vi "PageEngine.vi"() -> ()   [LabVIEW 2016, in "PCM PanelSplit.lvclass"]
uses:
  PCM PanelSplit.lvclass
  <vilib>/Utility/error.llb/DialogType.ctl
  PanelSplitToolkit/QueueManager.llb/CreatQueue.vi
  PanelSplitToolkit/QueueManager.llb/Remove.vi
  PanelSplitToolkit/QueueManager.llb/Insert.vi
  PanelSplitToolkit/QueueManager.llb/Destroy.vi
  PanelSplitToolkit/PanelRootNode/PanelRootNode.lvclass
panel:
  in  "Parameters":T1
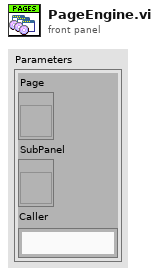
[diagram p1: front panel]
types:
  T1 = cluster{"Page":refnum<vi>, "SubPanel":refnum<vi>, "Caller":string}
  T2 = cluster{"error":errorcluster, "Event":string, "Data":variant, "Q_Local":string, "DyPageNames":string[], "DyPageVIRefs":refnum<vi>[], "PageTreeTags":string[], "CurrentPage":string, "PageVIPath":path, "PanelUIQName":string, "Send":cluster{"VI*ToSend":refnum<vi>, "EventToSend":string, "DataToSend":variant}, "PageCtr*":refnum<vi>, "SubPanel*":refnum<vi>, "Q_Caller":string, "FixedPages":cluster{"FixedPageNames":string[], "FixedPageVIRefs":refnum<vi>[]}}
  T3 = cluster{"Page":refnum<vi>, "SubPanel":refnum<vi>}
  T4 = typedef "DialogType.ctl" = u16
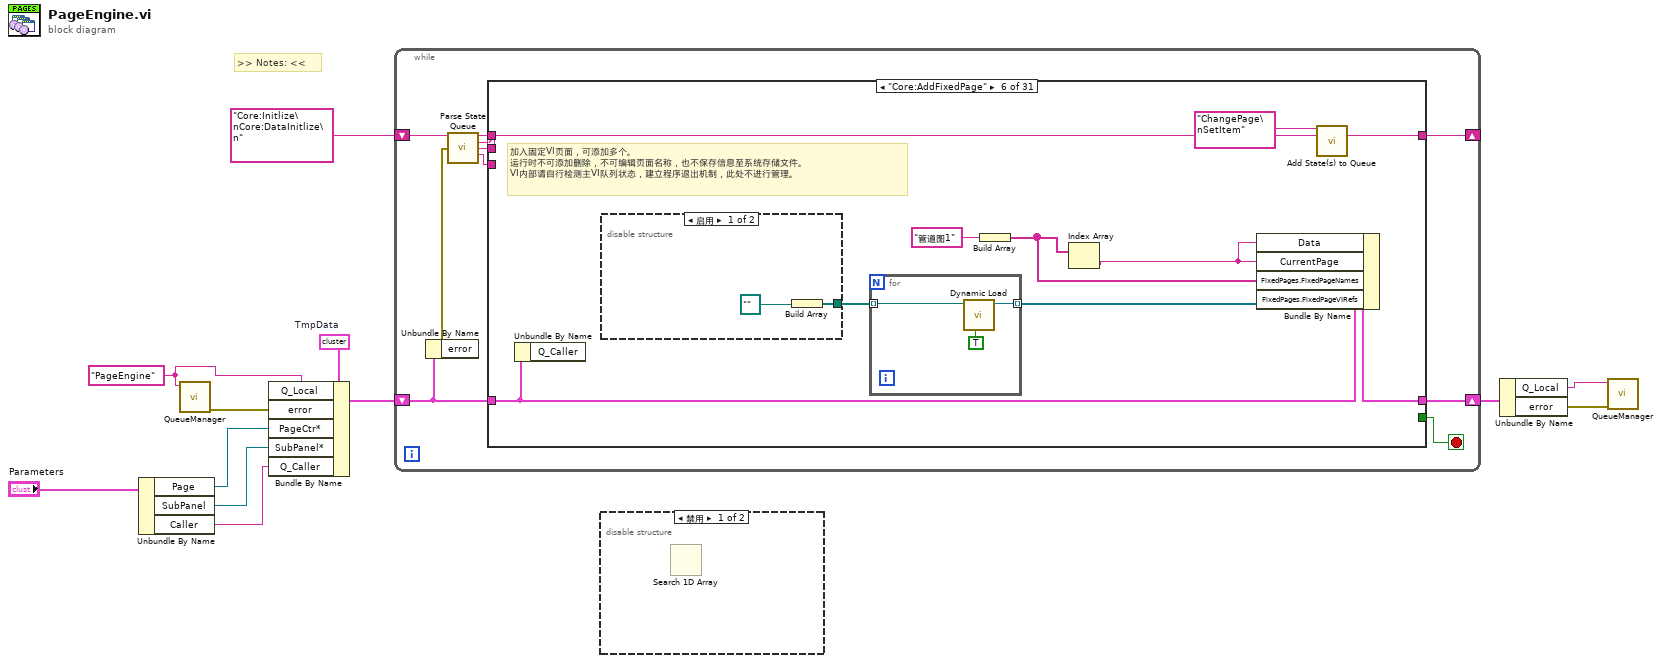
[diagram p0: block diagram]
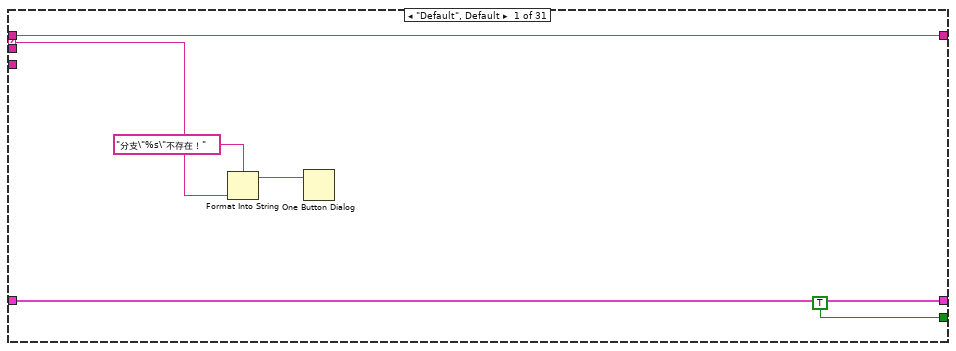
[diagram p3: hidden frame]
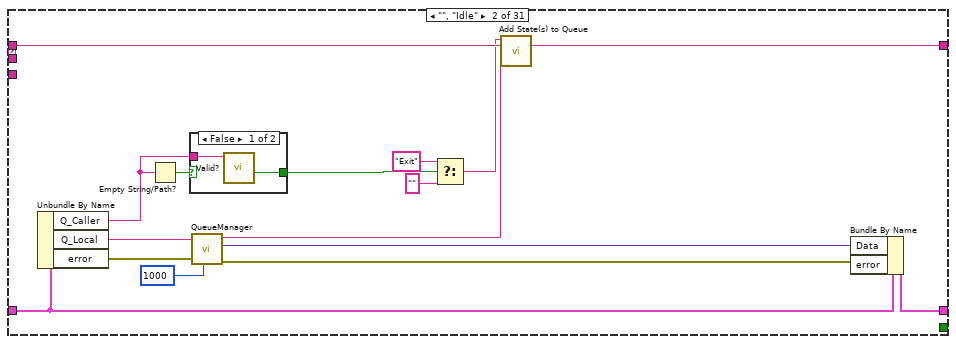
[diagram p4: hidden frame]
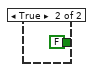
[diagram p5: hidden frame]
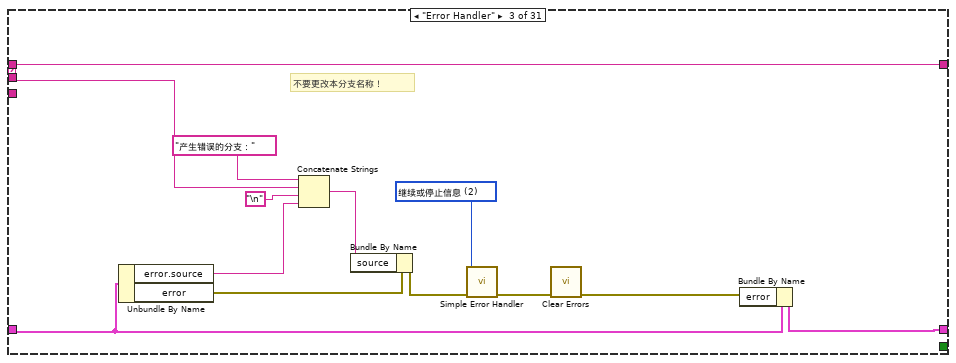
[diagram p6: hidden frame]
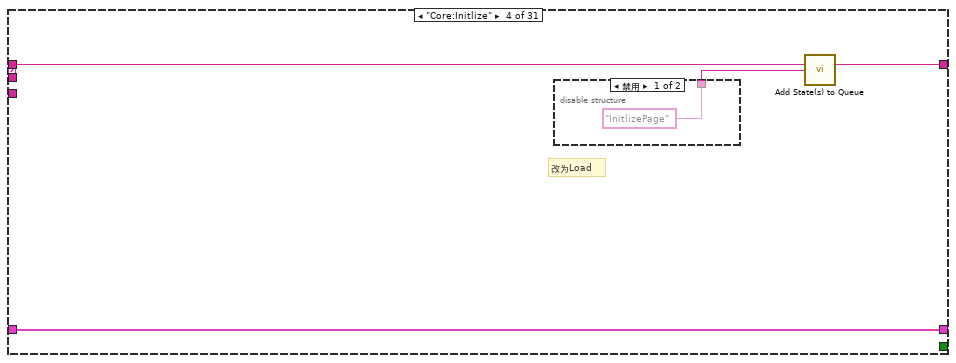
[diagram p7: hidden frame]
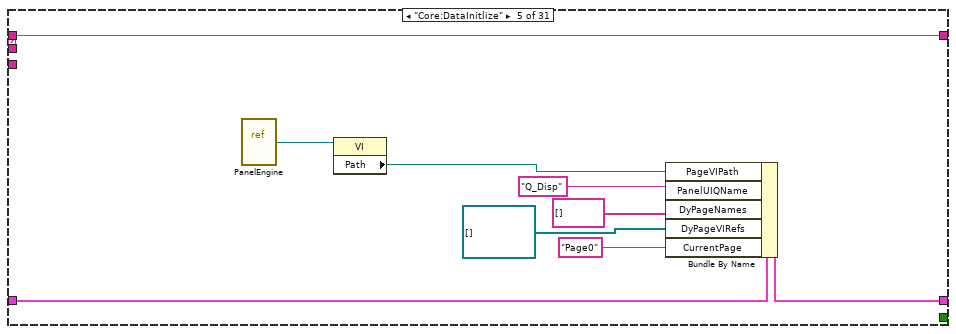
[diagram p9: hidden frame]
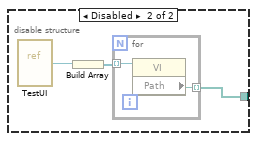
[diagram p10: hidden frame]
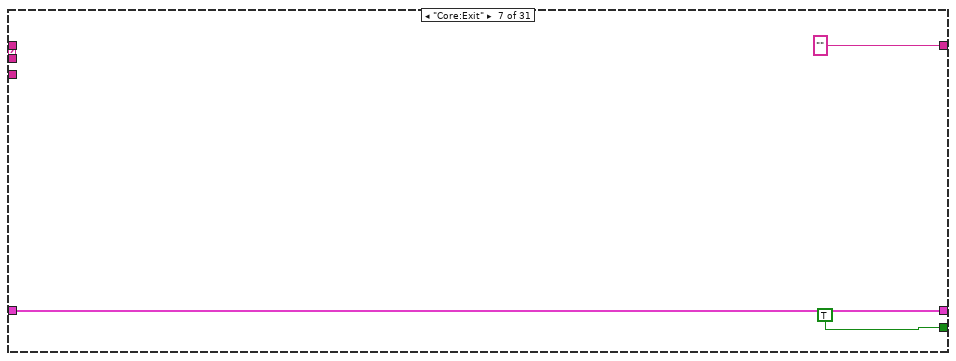
[diagram p11: hidden frame]
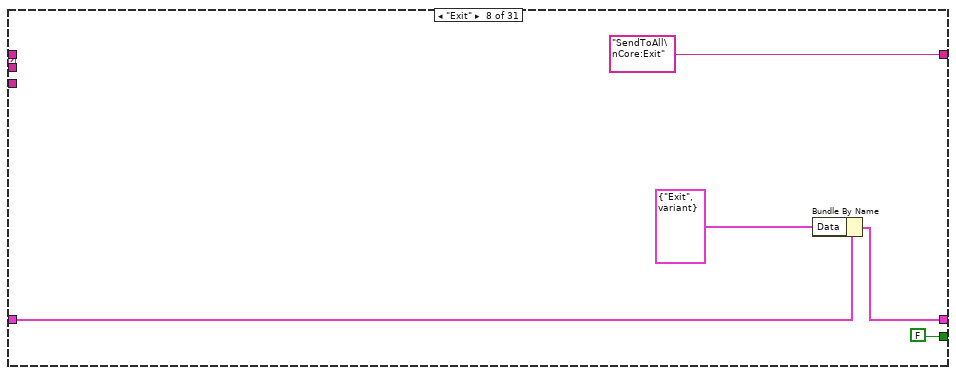
[diagram p12: hidden frame]
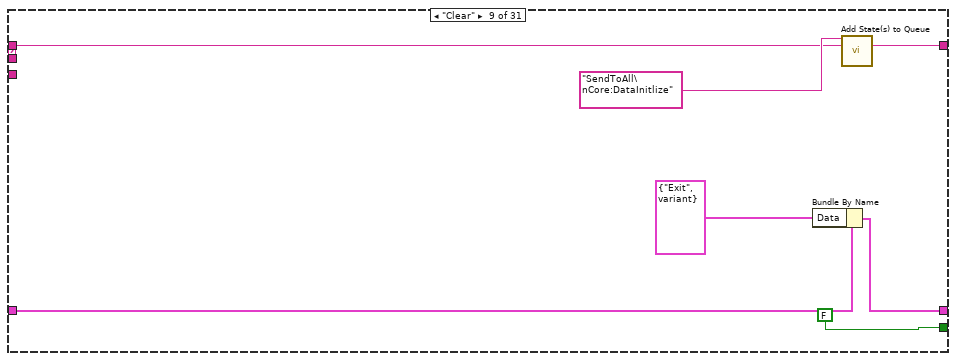
[diagram p13: hidden frame]
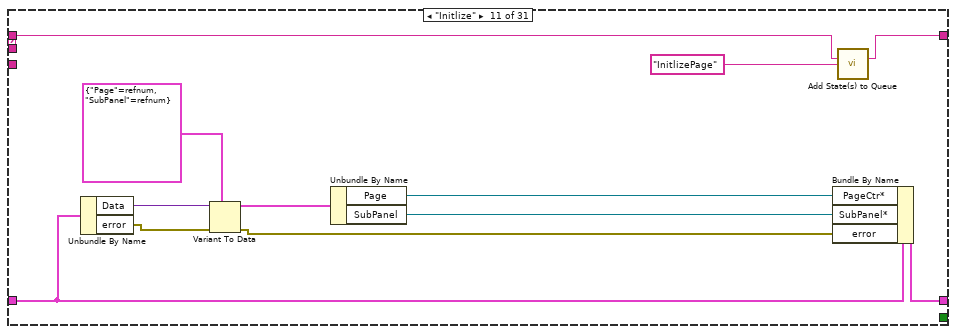
[diagram p15: hidden frame]
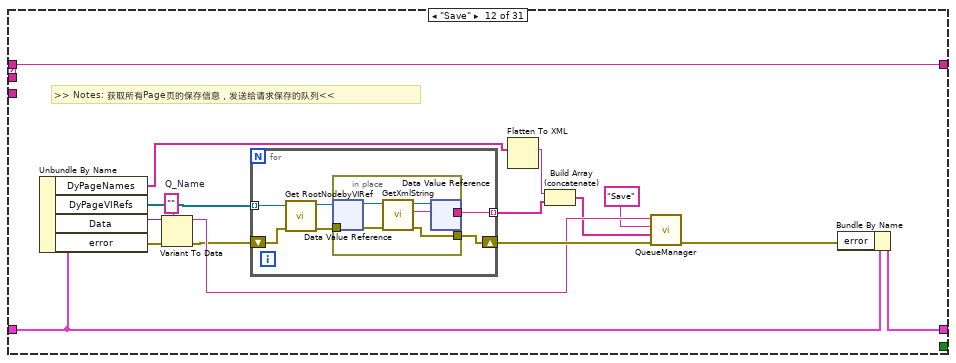
[diagram p16: hidden frame]
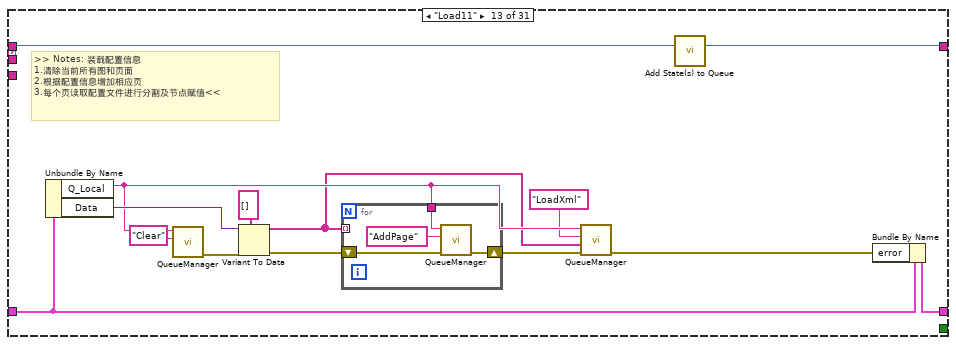
[diagram p17: hidden frame]
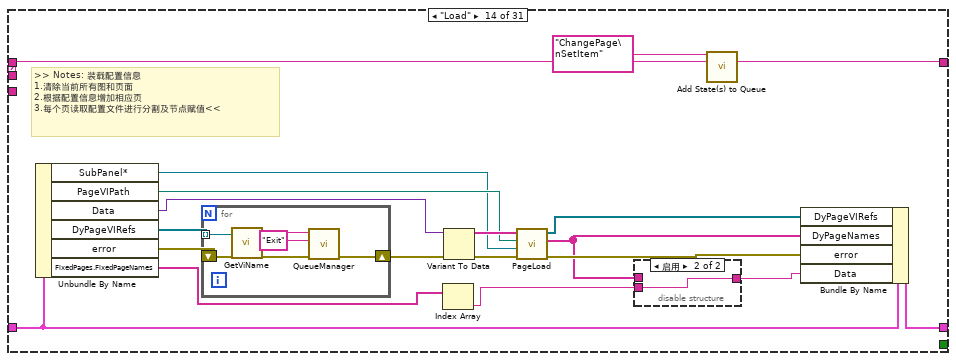
[diagram p18: hidden frame]
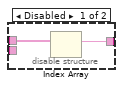
[diagram p19: hidden frame]
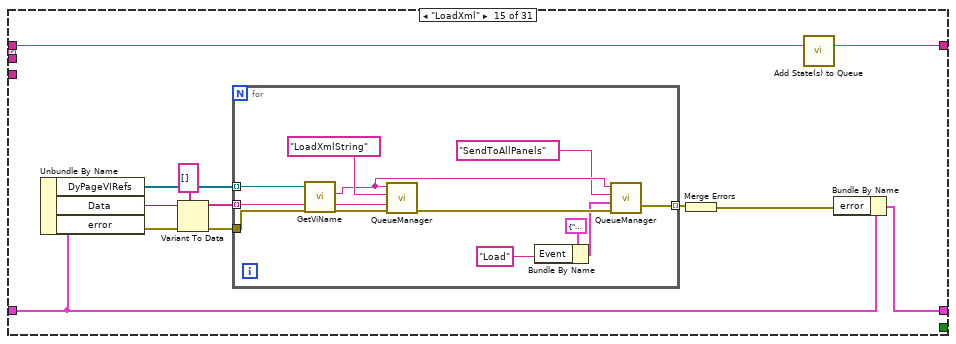
[diagram p20: hidden frame]
diagram:
  w9 = T2 {"error"={"status"=FALSE, "code"=0, "source"=""}, "Event"="", "Data"=variant, "Q_Local"="", "DyPageNames"=[], "DyPageVIRefs"=[], "PageTreeTags"=[], "CurrentPage"="", "PageVIPath"=path "", "PanelUIQName"="", "Send"={"VI*ToSend"=refnum, "EventToSend"="", "DataToSend"=variant}, "PageCtr*"=refnum, "SubPanel*"=refnum, "Q_Caller"="", "FixedPages"={"FixedPageNames"=[], "FixedPageVIRefs"=[]}}  # TmpData
  w7 = "PageEngine" ("QueueName")
  # ">> Notes: <<"
  n1 = Unbundle By Name("Parameters") -> ("Page"=w3:refnum<vi>, "SubPanel"=w2:refnum<vi>, "Caller"=w1:string)
  n2 = call-poly "QueueManager.vi"("QueueName"=w7) -> ("error out"=w5:errorcluster)  [unwired: 9 in, 1 out]
  n3 = Bundle By Name(cluster=w9, "Q_Local"=w7, "error"=w5, "PageCtr*"=w3, "SubPanel*"=w2, "Q_Caller"=w1) -> (w8:T2)
  n4 = while {
    shift-right: [w15] -> w10
    shift-left: w8 -> [w16]
    shift-right: [w14] -> _
    shift-left: "Core:Initlize\nCore:DataInitlize\n" -> [w22]
    stop <- w18 stop-if-true
    n5 = Unbundle By Name(w16) -> ("error"=w17:errorcluster)
    n6 = call "Parse State Queue.vi"("State Queue"=w22, "Error In (no error)"=w17) -> ("Remaining States"=w21:string, "Current State"=w20:string, "Arguments"=w19:string, "PreState"=w13:string)  [unwired: 10 in]
    n7 = case shown="\"Core:AddFixedPage\"" w20 {
      selector: w20 -> [w26 _ _ _ _ _ _ _ _ _ _ _ _ _ _ _ _ _ _ _ _ _ _ _ _ _ _ _ _ _ _]
      tunnel: w21 -> [w27 w40 w60 w63 w74 w78 _ _ w103 w111 w113 w139 w164 w187 w202 w221 w223 w228 w249 w277 w281 w290 w348 w350 w361 w372 w376 w397 w399 w411 w421]
      tunnel: w19 -> [_ _ w48 _ _ _ _ _ _ _ _ _ _ _ _ _ _ _ _ _ _ _ _ _ _ _ _ _ _ _ _]
      tunnel: [TRUE _ _ _ _ _ TRUE FALSE FALSE _ _ _ _ _ _ _ FALSE FALSE _ _ _ _ _ _ _ _ _ _ _ _ _] -> w18
      tunnel: w16 -> [w28 w37 w50 w64 w73 w76 w96 w99 w107 w110 w121 w137 w154 w185 w206 w222 w224 w229 w258 w272 w283 w292 w340 w349 w352 w363 w381 w392 w398 w402 w423]
      tunnel: [w28 w43 w49 w64 w72 w84 w96 w98 w106 w110 w120 w136 w152 w184 w205 w222 w224 w230 w256 w271 w282 w291 w339 w349 w351 w362 w377 w390 w398 w401 w418] -> w15
      tunnel: [w27 w39 w60 w62 w74 w77 "" ("Remaining States") "SendToAll\nCore:Exit" ("Remaining States") w104 w111 w112 w139 w163 w186 w201 w220 w223 w227 w248 w277 w280 w289 w348 w350 w361 w372 w375 w397 w399 w411 w420] -> w14
      tunnel: w13 -> [_ _ _ _ _ _ _ _ _ _ _ _ _ _ _ _ _ _ _ _ _ _ _ _ _ _ _ _ _ _ _]
      frame "Default", Default {
        n8 = Format Into String(format string="分支\"%s\"不存在！" ("格式字符串"), w26) -> (resulting string=w25:string)  [unwired: 2 in, 1 out]
        n9 = One Button Dialog(message=w25) -> ()  [unwired: 1 in, 1 out]
      }
      frame "", "Idle" {
        n10 = Unbundle By Name(w37) -> ("Q_Caller"=w30:string, "Q_Local"=w36:string, "error"=w35:errorcluster)
        n11 = Empty String/Path?(string/path=w30) -> (empty?=w34:bool)
        n12 = case shown="False" w34 {
          tunnel: [w46 FALSE ("Not Exist?")] -> w33
          tunnel: w30 -> [w45 _]
          frame False {
            n13 = call "Valid?.vi"("Queue Name(unamed)"=w45) -> ("Not Exist?"=w46:bool)  [unwired: 9 in, 1 out]
          }
          frame True {
          }
        }
        n14 = call-poly "QueueManager.vi"("Time out(-1)"=1000, "error in (no error)"=w35, "Queue Name"=w36) -> ("error out"=w44:errorcluster, "Data"=w42:variant, "Event"=w41:string)  [unwired: 5 in, 1 out]
        n15 = Select(t="Exit" ("Event"), s=w33, f="") -> (s? t:f=w29:string)
        n16 = call "Add State(s) to Queue.vi"("State(s) in Front (\"\")"=w29, "State(s) in (\"\")"=w40, "State(s) at Back (\"\")"=w41) -> ("States Out"=w39:string)  [unwired: 12 in]
        n17 = Bundle By Name(cluster=w37, "Data"=w42, "error"=w44) -> (w43:T2)
      }
      frame "Error Handler" {
        w57 = T4 2 items=["无对话框", "确定信息", "继续或停止信息", "确定信息＋警告", "继续/停止+警告"] ("type of dialog (OK msg:1)")
        # "不要更改本分支名称！"
        n18 = Unbundle By Name(w50) -> ("error.source"=w51:string, "error"=w53:errorcluster)
        n19 = Concatenate Strings("产生错误的分支：" ("字符串"), w48, "\n", w51) -> (w54:string)
        n20 = Bundle By Name(cluster=w53, "source"=w54) -> (w52:errorcluster)
        n21 = call <vilib>:"Simple Error Handler.vi"("type of dialog (OK msg:1)"=w57, "error in (no error)"=w52) -> ("error out"=w58:errorcluster)  [unwired: 3 in, 4 out]
        n22 = call <vilib>:"Clear Errors.vi"("error in (no error)"=w58) -> ("error out"=w59:errorcluster)  [unwired: 5 in, 1 out]
        n23 = Bundle By Name(cluster=w50, "error"=w59) -> (w49:T2)
      }
      frame "Core:Initlize" {
        # "改为Load"
        n24 = disable-structure shown="禁用" {
          disable-tunnel: ["InitlizePage" ("State(s) at Back (\"\")") _] -> w61
          frame Disabled {
          }
          frame Enabled {
          }
        }
        n25 = call "Add State(s) to Queue.vi"("State(s) in (\"\")"=w63, "State(s) at Back (\"\")"=w61) -> ("States Out"=w62:string)  [unwired: 13 in]
      }
      frame "Core:DataInitlize" {
        n26 = vi-ref "PanelEngine.vi"() -> (w70:refnum<vi>)
        n27 = property class="VI"(reference=w70) -> ("Path"=w69:path)  [unwired: 1 in, 2 out]
        n28 = Bundle By Name(cluster=w73, "PageVIPath"=w69, "PanelUIQName"="Q_Disp", "DyPageNames"=string[] [] ("PageNames"), "DyPageVIRefs"=refnum<vi>[] [] ("PageVIRefs"), "CurrentPage"="Page0") -> (w72:T2)
      }
      frame "Core:AddFixedPage" {
        # "加入固定VI页面，可添加多个。\n运行时不可添加删除，不可编辑页面名称，也不保存信息至系统存储文件。\nVI内部请自行检测主VI队列状态，建立程序退出机制，此处不进行管理。"
        n29 = Unbundle By Name(w76) -> ()  [unwired: 1 out]
        n30 = disable-structure shown="启用" {
          disable-tunnel: [w85 w89] -> w82
          frame Enabled {
            n31 = Build Array(path "" ("Vi Path")) -> (w85:path[])
          }
          frame Disabled {
            n32 = vi-ref "TestUI.vi"() -> (w87:refnum<vi>)
            n33 = Build Array(w87) -> (w88:refnum<vi>[])
            n34 = for {
              tunnel: w88 -> [w91] mode=indexing
              tunnel: [w90] -> w89 mode=indexing
              n35 = property class="VI"(reference=w91) -> ("Path"=w90:path)  [unwired: 1 in, 2 out]
            }
          }
        }
        n36 = for {
          tunnel: [w94] -> w83 mode=indexing
          tunnel: w82 -> [w93] mode=indexing
          n37 = call "Dynamic Load.vi"("Auto Dispose Ref"=TRUE, "Vi Path"=w93) -> ("vi reference"=w94:refnum<vi>)  [unwired: 8 in, 1 out]
        }
        n38 = Build Array("管道图1") -> (w80:string[])
        n39 = Index Array(array=w80) -> (element=w75:string)  [unwired: 1 in]
        n40 = Bundle By Name(cluster=w76, "Data"=w75, "CurrentPage"=w75, "FixedPages.FixedPageNames"=w80, "FixedPages.FixedPageVIRefs"=w83) -> (w84:T2)
        n41 = call "Add State(s) to Queue.vi"("State(s) in Front (\"\")"="ChangePage\nSetItem" ("State(s) in Front (\"\")"), "State(s) in (\"\")"=w78) -> ("States Out"=w77:string)  [unwired: 13 in]
      }
      frame "Core:Exit" {
      }
      frame "Exit" {
        n42 = Bundle By Name(cluster=w99, "Data"=cluster{string, "变体":variant} {"Exit", "变体"=variant}) -> (w98:T2)
      }
      frame "Clear" {
        n43 = Bundle By Name(cluster=w107, "Data"=cluster{string, "变体":variant} {"Exit", "变体"=variant}) -> (w106:T2)
        n44 = call "Add State(s) to Queue.vi"("State(s) in Front (\"\")"="SendToAll\nCore:DataInitlize" ("Remaining States"), "State(s) in (\"\")"=w103) -> ("States Out"=w104:string)  [unwired: 13 in]
      }
      frame "--------Init------------" {
      }
      frame "Initlize" {
        n45 = Unbundle By Name(w121) -> ("Data"=w123:variant, "error"=w115:errorcluster)
        n46 = Variant To Data(error in=w115, type=T3 {"Page"=refnum, "SubPanel"=refnum}, Variant=w123) -> (data=w119:T3, error out=w116:errorcluster)
        n47 = Unbundle By Name(w119) -> ("Page"=w118:refnum<vi>, "SubPanel"=w117:refnum<vi>)
        n48 = Bundle By Name(cluster=w121, "PageCtr*"=w118, "SubPanel*"=w117, "error"=w116) -> (w120:T2)
        n49 = call "Add State(s) to Queue.vi"("State(s) in (\"\")"=w113, "State(s) at Back (\"\")"="InitlizePage" ("State(s) in Front (\"\")")) -> ("States Out"=w112:string)  [unwired: 13 in]
      }
      frame "Save" {
        w134 = ""  # Q_Name
        # ">> Notes: 获取所有Page页的保存信息，发送给请求保存的队列<<"
        n50 = Unbundle By Name(w137) -> ("DyPageNames"=w125:string[], "DyPageVIRefs"=w138:refnum<vi>[], "Data"=w135:variant, "error"=w128:errorcluster)
        n51 = Variant To Data(error in=w128, type=w134, Variant=w135) -> (data=w131:string, error out=w129:errorcluster)
        n52 = for {
          tunnel: w138 -> [w143] mode=indexing
          tunnel: [w145] -> w127 mode=indexing
          shift-right: [w144] -> w133
          shift-left: w129 -> [w140]
          n53 = call "Get RootNodebyVIRef.vi"("error in"=w140, "vi*"=w143) -> ("error out"=w141:errorcluster, "RootNode*"=w142:refnum<data-value>)  [unwired: 8 in]
          n54 = in-place {
            in-place-border: w141 -> [w148]
            in-place-border: [w147] -> w144
            in-place-border: [w146] -> w145
            n55 = in-place-dvr #1(w142) -> (w150:refnum<class "PanelRootNode.lvclass">)  [unwired: 1 out]
            n56 = call-dynamic "GetXmlString.vi"("error in"=w148, "PanelRootNode 输入"=w150) -> ("error out"=w147:errorcluster, "XML"=w146:string, "PanelRootNode 输出"=w149:refnum<class "PanelRootNode.lvclass">)  [unwired: 7 in]
            n57 = in-place-dvr #1(w149) -> ()  [unwired: 2 out]
          }
        }
        n58 = Flatten To XML(anything=w125) -> (xml string=w124:string)
        n59 = Build Array (concatenate)(w124, w127) -> (w126:string[])
        n60 = call-poly "QueueManager.vi"("error in"=w133, "Data"=w126, "Event"="Save", "QueueName"=w131) -> ("error out"=w132:errorcluster)  [unwired: 6 in, 1 out]
        n61 = Bundle By Name(cluster=w137, "error"=w132) -> (w136:T2)
      }
      frame "Load11" {
        # ">> Notes: 装载配置信息\n1.清除当前所有图和页面\n2.根据配置信息增加相应页\n3.每个页读取配置文件进行分割及节点赋值<<"
        n62 = Unbundle By Name(w154) -> ("Q_Local"=w156:string, "Data"=w161:variant)
        n63 = call-poly "QueueManager.vi"("Event"="Clear", "QueueName"=w156) -> ("error out"=w159:errorcluster)  [unwired: 8 in, 1 out]
        n64 = Variant To Data(error in=w159, type=string[] [], Variant=w161) -> (data=w151:string[], error out=w158:errorcluster)
        n65 = for {
          tunnel: w156 -> [w167]
          tunnel: w151 -> [_] mode=indexing
          shift-right: [w165] -> w157
          shift-left: w158 -> [w168]
          n66 = call-poly "QueueManager.vi"("error in"=w168, "Event"="AddPage", "QueueName"=w167) -> ("error out"=w165:errorcluster)  [unwired: 7 in, 1 out]
        }
        n67 = call-poly "QueueManager.vi"("error in"=w157, "Data"=w151, "Event"="LoadXml", "QueueName"=w156) -> ("error out"=w153:errorcluster)  [unwired: 6 in, 1 out]
        n68 = call "Add State(s) to Queue.vi"("State(s) in (\"\")"=w164) -> ("States Out"=w163:string)  [unwired: 14 in]
        n69 = Bundle By Name(cluster=w154, "error"=w153) -> (w152:T2)
      }
      frame "Load" {
        # ">> Notes: 装载配置信息\n1.清除当前所有图和页面\n2.根据配置信息增加相应页\n3.每个页读取配置文件进行分割及节点赋值<<"
        n70 = Unbundle By Name(w185) -> ("SubPanel*"=w176:refnum<vi>, "PageVIPath"=w177:path, "Data"=w180:variant, "DyPageVIRefs"=w183:refnum<vi>[], "error"=w182:errorcluster, "FixedPages.FixedPageNames"=w170:string[])
        n71 = for {
          tunnel: w183 -> [w195] mode=indexing
          shift-right: [w193] -> w181
          shift-left: w182 -> [w192]
          n72 = call "GetViName.vi"("VI*"=w195) -> ("VI Name"=w194:string)  [unwired: 9 in, 1 out]
          n73 = call-poly "QueueManager.vi"("error in"=w192, "Event"="Exit", "QueueName"=w194) -> ("error out"=w193:errorcluster)  [unwired: 7 in, 1 out]
        }
        n74 = Index Array(array=w170) -> (element=w169:string)  [unwired: 1 in]
        n75 = Variant To Data(error in=w181, Variant=w180) -> (data=w178:string[], error out=w179:errorcluster)  [unwired: 1 in]
        n76 = call "PageLoad.vi"("error in"=w179, "SubPanel*"=w176, "PanelVIPath"=w177, "data"=w178) -> ("error out"=w174:errorcluster, "PageNames"=w173:string[], "VIRefs"=w175:refnum<vi>[])  [unwired: 5 in]
        n77 = disable-structure shown="启用" {
          disable-tunnel: w173 -> [w189 _]
          disable-tunnel: [w188 w190] -> w172
          disable-tunnel: w169 -> [_ w190]
          frame Disabled {
            n78 = Index Array(array=w189) -> (element=w188:string)  [unwired: 1 in]
          }
          frame Enabled {
          }
        }
        n79 = call "Add State(s) to Queue.vi"("State(s) in Front (\"\")"="ChangePage\nSetItem" ("State(s) in Front (\"\")"), "State(s) in (\"\")"=w187) -> ("States Out"=w186:string)  [unwired: 13 in]
        n80 = Bundle By Name(cluster=w185, "DyPageVIRefs"=w175, "DyPageNames"=w173, "error"=w174, "Data"=w172) -> (w184:T2)
      }
      frame "LoadXml" {
        n81 = Unbundle By Name(w206) -> ("DyPageVIRefs"=w207:refnum<vi>[], "Data"=w200:variant, "error"=w196:errorcluster)
        n82 = Variant To Data(error in=w196, type=string[] [], Variant=w200) -> (data=w199:string[], error out=w197:errorcluster)
        n83 = for {
          tunnel: w207 -> [w218] mode=indexing
          tunnel: w199 -> [w217] mode=indexing
          tunnel: [w214] -> w204 mode=indexing
          tunnel: w197 -> [w208]
          n84 = call "GetViName.vi"("VI*"=w218) -> ("VI Name"=w213:string)  [unwired: 9 in, 1 out]
          n85 = call-poly "QueueManager.vi"("error in"=w208, "Data"=w217, "Event"="LoadXmlString", "QueueName"=w213) -> ("error out"=w215:errorcluster)  [unwired: 6 in, 1 out]
          n86 = Bundle By Name(cluster=cluster{"Event":string, "Data":variant} {"Event"="", "Data"=variant} ("Send"), "Event"="Load") -> (w210:cluster{"Event":string, "Data":variant})
          n87 = call-poly "QueueManager.vi"("error in"=w215, "Data"=w210, "Event"="SendToAllPanels", "QueueName"=w213) -> ("error out"=w214:errorcluster)  [unwired: 6 in, 1 out]
        }
        n88 = Merge Errors(w204) -> (w203:errorcluster)
        n89 = call "Add State(s) to Queue.vi"("State(s) in (\"\")"=w202) -> ("States Out"=w201:string)  [unwired: 14 in]
        n90 = Bundle By Name(cluster=w206, "error"=w203) -> (w205:T2)
      }
      frame "New" {
        # ">> Notes: 响应主程序的“新建”指令，清除所有页面，然后加载一个波形图表<<"
        n91 = call "Add State(s) to Queue.vi"("State(s) in (\"\")"=w221, "State(s) at Back (\"\")"="Clear\nAddPage" ("State(s) at Back (\"\")")) -> ("States Out"=w220:string)  [unwired: 13 in]
      }
      frame "-----PageManager------" {
      }
      frame "InitlizePage" {
        n92 = disable-structure shown="禁用" {
          disable-tunnel: [w242 w243] -> w230
          disable-tunnel: w229 -> [w241 w243]
          disable-tunnel: ["ChangePage" ("State(s) in Front (\"\")") "AddPage" ("State(s) in Front (\"\")")] -> w226
          frame Disabled {
            w234 = "Page0" ("CurrentPage")
            n93 = Unbundle By Name(w241) -> ("PageVIPath"=w240:path, "error"=w238:errorcluster)
            n94 = call "Dynamic Load.vi"("Auto Dispose Ref"=TRUE ("自动销毁引用"), "error in"=w238, "Vi Path"=w240) -> ("错误输出"=w235:errorcluster, "vi reference"=w239:refnum<vi>)  [unwired: 7 in]
            n95 = Build Array(w239) -> (w237:refnum<vi>[])
            n96 = Build Array(w234) -> (w236:string[])
            n97 = Bundle By Name(cluster=w241, "CurrentPage"=w234, "DyPageNames"=w236, "DyPageVIRefs"=w237, "error"=w235, "Data"=w234) -> (w242:T2)
          }
          frame Enabled {
          }
        }
        n98 = call "Add State(s) to Queue.vi"("State(s) in Front (\"\")"=w226, "State(s) in (\"\")"=w228) -> ("States Out"=w227:string)  [unwired: 13 in]
      }
      frame "AddPage" {
        n99 = Unbundle By Name(w258) -> ("DyPageVIRefs"=w254:refnum<vi>[], "PageVIPath"=w255:path, "DyPageNames"=w246:string[])
        n100 = for {
          N: 100 -> [_]
          tunnel: w246 -> [w264]
          tunnel: "Page" -> [w267]
          tunnel: [w261] -> w250
          i -> [w266]
          stop <- w262 stop-if-true
          n101 = Number To Decimal String(number=w266) -> (decimal integer string=w265:string)  [unwired: 1 in]
          n102 = Concatenate Strings(w267, w265) -> (w261:string)
          n103 = Search 1D Array(1D array=w264, element=w261) -> (index of element=w263:i32)  [unwired: 1 in]
          n104 = Less Than 0?(x=w263) -> (x < 0?=w262:bool)
        }
        n105 = call "Dynamic Load.vi"("Auto Dispose Ref"=TRUE ("自动销毁引用"), "Vi Path"=w255) -> ("错误输出"=w252:errorcluster, "vi reference"=w253:refnum<vi>)  [unwired: 8 in]
        n106 = Build Array (concatenate)(w246, w250) -> (w257:string[])
        n107 = Build Array (concatenate)(w254, w253) -> (w251:refnum<vi>[])
        n108 = Bundle By Name(cluster=w258, "DyPageVIRefs"=w251, "error"=w252, "DyPageNames"=w257, "Data"=w250) -> (w256:T2)
        n109 = call "Add State(s) to Queue.vi"("State(s) in Front (\"\")"="ChangePage\nSetItem" ("State(s) in Front (\"\")"), "State(s) in (\"\")"=w249) -> ("States Out"=w248:string)  [unwired: 13 in]
      }
      frame "SetItem" {
        n110 = Unbundle By Name(w272) -> ("FixedPages.FixedPageNames"=w270:string[], "DyPageNames"=w269:string[], "PageCtr*"=w276:refnum<vi>, "CurrentPage"=w275:string)
        n111 = Build Array (concatenate)(w270, w269) -> (w268:string[])
        n112 = Search 1D Array(1D array=w268, element=w275) -> (index of element=w274:i32)  [unwired: 1 in]
        n113 = property class="Ring"(reference=w276, "Strings []"=w268, "Value"=w274) -> (error out=w273:errorcluster)  [unwired: 1 in, 1 out]
        n114 = Bundle By Name(cluster=w272, "error"=w273) -> (w271:T2)
      }
      frame "EditPageNames" {
        n115 = Unbundle By Name(w283) -> ("DyPageNames"=w279:string[], "PageCtr*"=w285:refnum<vi>)
        n116 = call "EditPageNames UI.vi"("PageNames"=w279) -> ("PageNames out"=w278:string[])  [unwired: 10 in]
        n117 = property class="Ring"(reference=w285, "Strings []"=w278) -> (error out=w284:errorcluster)  [unwired: 1 in, 1 out]
        n118 = Bundle By Name(cluster=w283, "DyPageNames"=w278, "error"=w284) -> (w282:T2)
        n119 = call "Add State(s) to Queue.vi"("State(s) in (\"\")"=w281) -> ("States Out"=w280:string)  [unwired: 14 in]
      }
      frame "DeletePage" {
        n120 = Unbundle By Name(w292) -> ("DyPageVIRefs"=w293:refnum<vi>[], "DyPageNames"=w288:string[], "CurrentPage"=w287:string)
        n121 = Search 1D Array(1D array=w288, element=w287) -> (index of element=w286:i32)  [unwired: 1 in]
        n122 = case shown="0, Default" w286 {
          tunnel: w293 -> [_ w310]
          tunnel: w292 -> [w296 w309]
          tunnel: [w296 w306] -> w291
          tunnel: w290 -> [w295 w304]
          tunnel: [w295 w303] -> w289
          tunnel: w288 -> [_ w298]
          tunnel: w287 -> [_ w297]
          frame -1 {
            n123 = One Button Dialog(message="该页面不允许删除！" ("消息")) -> ()  [unwired: 1 in, 1 out]
          }
          frame 0, Default {
            n124 = Array Size(array=w298) -> (size(s)=w305:i32)
            n125 = case shown="2.., Default" w305 {
              tunnel: w297 -> [w324 w327]
              tunnel: w310 -> [w322 w329]
              tunnel: [w318 w330] -> w308
              tunnel: [w320 w329] -> w307
              tunnel: w298 -> [w319 w330]
              tunnel: [w317 w327] -> w302
              tunnel: ["ChangePage\nSendToSingle\nSetItem" ("State(s) in Front (\"\")") "" ("State(s) in Front (\"\")")] -> w301
              tunnel: [w312 refnum<vi> refnum ("VI引用")] -> w300
              tunnel: ["Exit" ""] -> w299
              frame 2.., Default {
                # "删除页名、VI引用，切换到页面、关闭删除的VI、删除控件对应项"
                # "切换到第0页"
                n126 = Search 1D Array(1D array=w319, element=w324) -> (index of element=w315:i32)  [unwired: 1 in]
                n127 = Delete From Array(array=w319, length=1 ("长度"), index=w315) -> (array with subset deleted=w318:string[])  [unwired: 1 out]
                n128 = Delete From Array(array=w322, length=1 ("长度"), index=w315) -> (deleted portion=w313:refnum<vi>[], array with subset deleted=w320:refnum<vi>[])
                n129 = Index Array(array=w313) -> (element=w312:refnum<vi>)  [unwired: 1 in]
                n130 = Index Array(array=w318, index=0 ("索引")) -> (element=w317:string)
              }
              frame 1 {
                # "只有一页时不允许删"
              }
            }
            n131 = Bundle By Name(cluster=w309, "DyPageNames"=w308, "DyPageVIRefs"=w307, "Data"=w302, "Send.VI*ToSend"=w300, "Send.EventToSend"=w299) -> (w306:T2)
            n132 = call "Add State(s) to Queue.vi"("State(s) in Front (\"\")"=w301, "State(s) in (\"\")"=w304) -> ("States Out"=w303:string)  [unwired: 13 in]
          }
        }
      }
      frame "ChangePage" {
        n133 = Unbundle By Name(w340) -> ("SubPanel*"=w337:refnum<vi>, "FixedPages.FixedPageVIRefs"=w333:refnum<vi>[], "DyPageVIRefs"=w332:refnum<vi>[], "FixedPages.FixedPageNames"=w336:string[], "DyPageNames"=w335:string[], "Data"=w347:variant, "error"=w346:errorcluster)
        n134 = Variant To Data(error in=w346, type="" ("PageName"), Variant=w347) -> (data=w338:string, error out=w342:errorcluster)
        n135 = Build Array (concatenate)(w333, w332) -> (w331:refnum<vi>[])
        n136 = Build Array (concatenate)(w336, w335) -> (w334:string[])
        n137 = Search 1D Array(1D array=w334, element=w338) -> (index of element=w344:i32)  [unwired: 1 in]
        n138 = Index Array(array=w331, index=w344) -> (element=w343:refnum<vi>)
        n139 = invoke class="SubPnl" method="Insert VI"(reference=w337, error in=w342, "VI Ref"=w343) -> (error out=w341:errorcluster)  [unwired: 1 in, 3 out]
        n140 = Bundle By Name(cluster=w340, "error"=w341, "CurrentPage"=w338) -> (w339:T2)
      }
      frame "-----PanelManager------" {
      }
      frame "AddPanel" {
        n141 = Unbundle By Name(w352) -> ("DyPageVIRefs"=w358:refnum<vi>[], "DyPageNames"=w359:string[], "CurrentPage"=w360:string)
        n142 = Search 1D Array(1D array=w359, element=w360) -> (index of element=w357:i32)  [unwired: 1 in]
        n143 = Index Array(array=w358, index=w357) -> (element=w356:refnum<vi>)
        n144 = call "GetViName.vi"("VI*"=w356) -> ("VI Name"=w355:string)  [unwired: 9 in, 1 out]
        n145 = call-poly "QueueManager.vi"("Event"="AddPanel", "QueueName"=w355) -> ("error out"=w353:errorcluster)  [unwired: 8 in, 1 out]
        n146 = Bundle By Name(cluster=w352, "error"=w353) -> (w351:T2)
      }
      frame "DeletePanel" {
        n147 = Unbundle By Name(w363) -> ("DyPageVIRefs"=w369:refnum<vi>[], "DyPageNames"=w370:string[], "CurrentPage"=w371:string)
        n148 = Search 1D Array(1D array=w370, element=w371) -> (index of element=w368:i32)  [unwired: 1 in]
        n149 = Index Array(array=w369, index=w368) -> (element=w367:refnum<vi>)
        n150 = call "GetViName.vi"("VI*"=w367) -> ("VI Name"=w366:string)  [unwired: 9 in, 1 out]
        n151 = call-poly "QueueManager.vi"("Event"="DeletePanel", "QueueName"=w366) -> ("error out"=w364:errorcluster)  [unwired: 8 in, 1 out]
        n152 = Bundle By Name(cluster=w363, "error"=w364) -> (w362:T2)
      }
      frame "TransferToSingle" {
        # "转发给当前PAGE的Panel引擎"
        n153 = Unbundle By Name(w381) -> ("DyPageVIRefs"=w383:refnum<vi>[], "DyPageNames"=w384:string[], "CurrentPage"=w385:string)
        n154 = Unbundle By Name(w381) -> ("Data"=w388:variant)
        n155 = Variant To Data(type=cluster{"Event":string, "Data":variant} {"Event"="", "Data"=variant}, Variant=w388) -> (data=w386:cluster{"Event":string, "Data":variant}, error out=w373:errorcluster)  [unwired: 1 in]
        n156 = Search 1D Array(1D array=w384, element=w385) -> (index of element=w382:i32)  [unwired: 1 in]
        n157 = Unbundle By Name(w386) -> ("Event"=w379:string, "Data"=w380:variant)
        n158 = Index Array(array=w383, index=w382) -> (element=w378:refnum<vi>)
        n159 = Bundle By Name(cluster=w381, "Send.VI*ToSend"=w378, "Send.EventToSend"=w379, "Send.DataToSend"=w380, "error"=w373) -> (w377:T2)
        n160 = call "Add State(s) to Queue.vi"("State(s) in Front (\"\")"="SendToSingle" ("State(s) in Front (\"\")"), "State(s) in (\"\")"=w376) -> ("States Out"=w375:string)  [unwired: 13 in]
      }
      frame "SendToSingle" {
        n161 = Unbundle By Name(w392) -> ("Send.EventToSend"=w393:string, "Send.DataToSend"=w394:variant, "Send.VI*ToSend"=w395:refnum<vi>, "error"=w389:errorcluster)
        n162 = call "GetViName.vi"("VI*"=w395) -> ("VI Name"=w396:string)  [unwired: 9 in, 1 out]
        n163 = call-poly "QueueManager.vi"("error in"=w389, "Data"=w394, "Event"=w393, "QueueName"=w396) -> ("error out"=w391:errorcluster)  [unwired: 6 in, 1 out]
        n164 = Bundle By Name(cluster=w392, "error"=w391) -> (w390:T2)
      }
      frame "--------Send----------" {
      }
      frame "SendToAll" {
        # ">> Notes: 发送给所有PanelEngine，不是发送给所有叶子节点面板<<"
        n165 = Unbundle By Name(w402) -> ("DyPageVIRefs"=w410:refnum<vi>[], "Data"=w409:variant, "error"=w404:errorcluster)
        n166 = Variant To Data(error in=w404, type=cluster{string, "Data":variant} {"", "Data"=variant}, Variant=w409) -> (data=w407:cluster{string, "Data":variant}, error out=w403:errorcluster)
        n167 = Unbundle(w407) -> (w406:string, "Data"=w405:variant)
        n168 = for {
          tunnel: w410 -> [w417] mode=indexing
          tunnel: w406 -> [w415]
          tunnel: w405 -> [w414]
          shift-right: [w413] -> w400
          shift-left: w403 -> [w412]
          n169 = call "GetViName.vi"("VI*"=w417) -> ("VI Name"=w416:string)  [unwired: 9 in, 1 out]
          n170 = call-poly "QueueManager.vi"("error in"=w412, "Data"=w414, "Event"=w415, "QueueName"=w416) -> ("error out"=w413:errorcluster)  [unwired: 6 in, 1 out]
        }
        n171 = Bundle By Name(cluster=w402, "error"=w400) -> (w401:T2)
      }
      frame "SendToAllPanels" {
        (unwired) cluster{"Event":string, "Data":variant} {"Event"="", "Data"=variant} ("Send")
        # ">> Notes: 发送至所有Page页的所有面板，变体Data的数据结构为包含字符串和变体的簇<<"
        n172 = Unbundle By Name(w423) -> ("Data"=w425:variant)
        n173 = disable-structure shown="\"调用形式如下\"" {
          frame condition #0 {
            n174 = call-poly "QueueManager.vi"("Data"=cluster{"Event":string, "Data":variant} {"Event"="", "Data"=variant} ("Send"), "Event"="SendToAllPanels", "QueueName"="PageEngine") -> ()  [unwired: 7 in, 2 out]
          }
          frame condition #1 (active) {
          }
        }
        n175 = Bundle("SendToAllPanels", "Data"=w425) -> (w422:cluster{string, "Data":variant})  [unwired: 1 in]
        n176 = Bundle By Name(cluster=w423, "Data"=w422) -> (w418:T2)
        n177 = call "Add State(s) to Queue.vi"("State(s) in Front (\"\")"="SendToAll" ("State(s) in Front (\"\")"), "State(s) in (\"\")"=w421) -> ("States Out"=w420:string)  [unwired: 13 in]
      }
    }
  }
  n178 = disable-structure shown="禁用" {
    frame Disabled {
      n179 = Search 1D Array() -> ()  [unwired: 3 in, 1 out]
    }
    frame Enabled {
    }
  }
  n180 = Unbundle By Name(w10) -> ("Q_Local"=w6:string, "error"=w11:errorcluster)
  n181 = call-poly "QueueManager.vi"("error in (no error)"=w11, "QueeuName"=w6) -> ()  [unwired: 9 in, 1 out]
